vi "Vehicle Position Simulation View.vi"(8 "error in (no error)":errorcluster, 11 "View Model":T1) -> (0 "error out":errorcluster, 3 "View Model":T1)   [LabVIEW 2017]
doc: "Generates Position Change event for CarWash Controller"
uses:
  View Model/Controls/View Model.ctl
  Configuration Database/Controls/Config Model.ctl
  Configuration Database/Controls/Congif Data.ctl
  Configuration Database/Controls/Config Commands.ctl
  View Model/Controls/Shared Model.ctl
  Error Handler/Controls/Error Model.ctl
  Error Handler/Controls/Error Data.ctl
  Error Handler/Controls/Error Type.ctl
  Car Wash Controller/Controls/Car Wash Model.ctl
  Car Wash Controller/Controls/Car Wash States.ctl
  Car Wash Controller/Controls/Controller Overhead.ctl
  Car Wash Controller/Controls/Vehicle Location.ctl
  Car Wash Controller/Controls/CarWash CMD.ctl
panel:
  in  "Vehicle Position Simulation":u8(slide) scale=0.0..4.0
  # "[Covers: UI4]"
  # "[Covers: UI4A]"
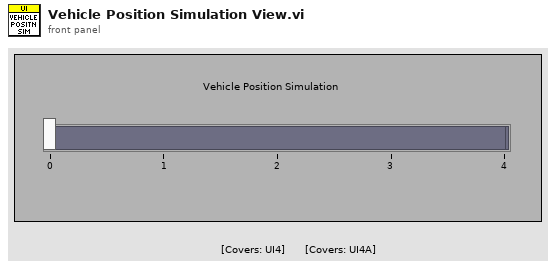
[diagram p1: front panel]
types:
  T1 = typedef "View Model.ctl" = cluster{"Config Model":T2, "Shared Model":T3, "Error Model":T4, "Car Wash Model":T5}
  T2 = typedef "Config Model.ctl" = cluster{"Config Event":refnum<user-event>, "Config DVR":refnum<data-value>, "Config CMD":refnum<user-event>, "Config Locked?":refnum<data-value>}
  T3 = typedef "Shared Model.ctl" = cluster{"Stop event":refnum<user-event>, "Stop DVR":refnum<data-value>}
  T4 = typedef "Error Model.ctl" = cluster{"Error event":refnum<user-event>, "Error DVR":refnum<data-value>}
  T5 = typedef "Car Wash Model.ctl" = cluster{"State Change":refnum<user-event>, "Out of Position Change":refnum<user-event>, "Wash Entry Change":refnum<user-event>, "Contr Overhead DVR":refnum<data-value>, "Contr Overhead Event":refnum<user-event>, "CarWash CMD":refnum<user-event>, "Location Change":refnum<user-event>}
  T6 = typedef "Vehicle Location.ctl" = enum16{"Entry", "Station 1", "Station 2", "Station 3", "Exit"}
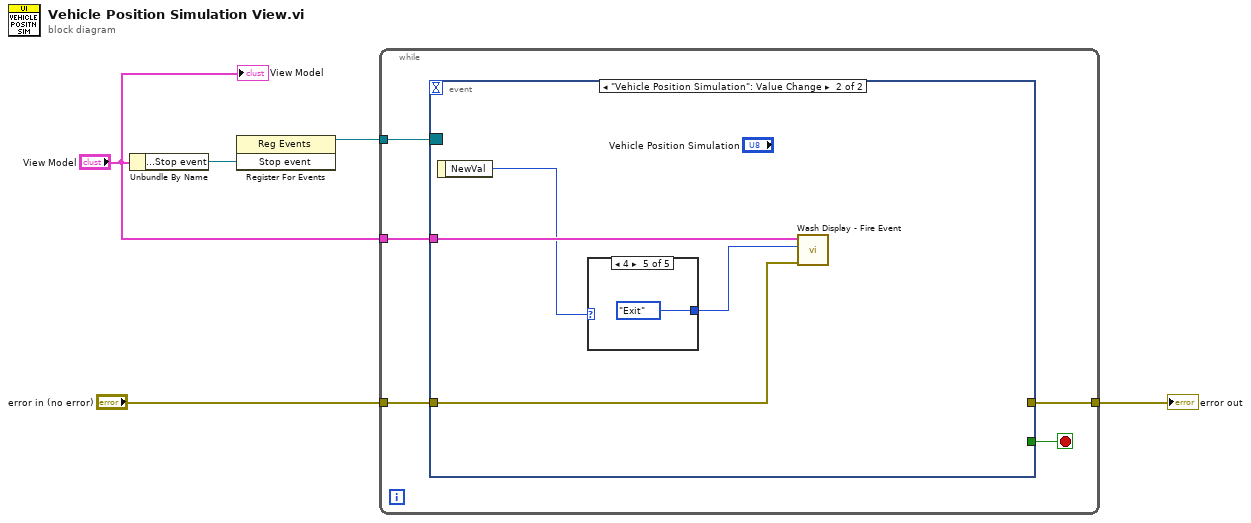
[diagram p0: block diagram]
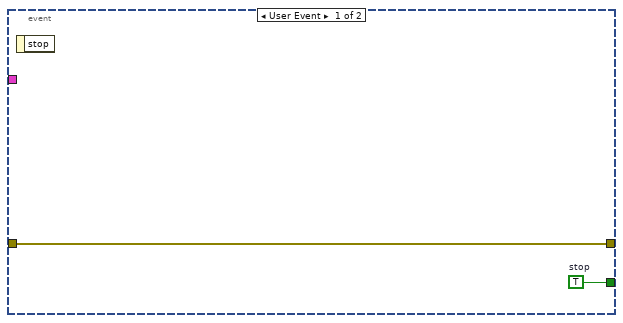
[diagram p2: hidden frame]
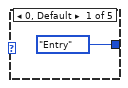
[diagram p3: hidden frame]
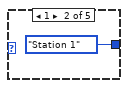
[diagram p4: hidden frame]
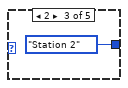
[diagram p5: hidden frame]
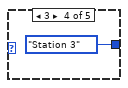
[diagram p6: hidden frame]
diagram:
  n1 = Unbundle By Name("View Model") -> ("Shared Model.Stop event"=w2:refnum<user-event>)
  n2 = register-events(w2) -> (reference out=w5:refnum<event-registration>)  [unwired: 2 in, 1 out]
  n3 = while {
    tunnel: w5 -> [w10]
    tunnel: "error in (no error)" -> [w8]
    tunnel: [w7] -> w3
    tunnel: "View Model" -> [w6]
    stop <- w9 stop-if-true
    n4 = event shown="[1] \"Vehicle Position Simulation\": Value Change" {
      selector: w10 -> [_ _]
      dyn-events: _ -> [_ _]
      timeout: _ -> [_ _]
      tunnel: [w12 _] -> w9
      tunnel: w8 -> [w11 w13]
      tunnel: [w11 _] -> w7
      tunnel: w6 -> [_ w16]
      event User Event {
        w12 = TRUE  # stop
        n5 = event-data() -> ()  [unwired: 1 in, 1 out]
      }
      event "Vehicle Position Simulation": Value Change {
        n6 = event-data() -> ("NewVal"=w15:u8)  [unwired: 1 in]
        n7 = case shown="4" w15 {
          tunnel: [Vehicle_Location."Entry" ("Location") Vehicle_Location."Station 1" ("Location") Vehicle_Location."Station 2" ("Location") Vehicle_Location."Station 3" ("Location") Vehicle_Location."Exit" ("Location")] -> w14
          frame 0, Default {
          }
          frame 1 {
          }
          frame 2 {
          }
          frame 3 {
          }
          frame 4 {
          }
        }
        n8 = call "Wash Display - Fire Event.vi"("error in (no error)"=w13, "Location"=w14, "View Model"=w16) -> ()  [unwired: 7 in, 2 out]
      }
    }
  }
  "error out" <- w3
  "View Model" <- "View Model"
